vi "ROI group-Remove ROI group.vi"(8 "error in (no error)":errorcluster) -> (0 "error out":errorcluster, 2 "Deleted group setup":T1={"Group number"="", "Group Name"="", "Visibility"=TRUE, "Highlight"=FALSE})   [LabVIEW 2020]
uses:
  Typedefs/Group sel cluster.ctl
  Global variables/gl_Functional Imaging-Global variables.vi
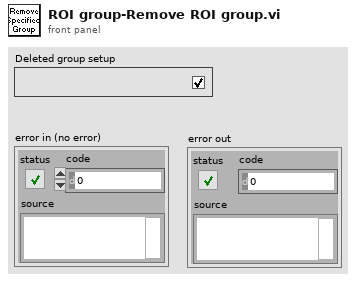
[diagram p1: front panel]
types:
  T1 = typedef "Group sel cluster.ctl" = cluster{"Group number":string, "Group Name":string, "Visibility":bool, "Highlight":bool}
  T2 = typedef "Functional Imging UI Refs.ctl" = cluster{"Menu ref":refnum<k9>, "Image control":refnum<vi>, "VI ref":refnum<vi>, "XGrapher":refnum<vi>, "Smoothing":refnum<vi>, "POI Averaging":refnum<vi>, "Normalize":refnum<vi>, "POI data points in each trial":refnum<vi>, "Channel":refnum<vi>, "Experiment data folder path":refnum<vi>, "[ROI vis]":refnum<vi>, "[Groups] visbl":T3, "Group Name":refnum<vi>, "POI index":refnum<vi>, "Trial No.":refnum<vi>, "Intensity Zoom":refnum<vi>, "Trial Cursor Enabled":refnum<vi>, "Number of Trials (ind 1)":refnum<vi>, "Number of Trials (ind 2)":refnum<vi>, "MiniScans Available":refnum<vi>, "POI Available":refnum<vi>, "Defer graph updates":refnum<vi>, "Waveform selector":refnum<vi>, "#of selected POI":refnum<vi>, "#of selected MiniScans":refnum<vi>, "#of selected groups":refnum<vi>, "Max Z-Projection":refnum<vi>, "Z-Plane Selector":refnum<vi>, "Index of miniscan point to visualise":refnum<vi>, "ROI vis. mode":refnum<vi>, "Total # of points":refnum<vi>, "Index of group clicked on":refnum<vi>, "Pane 1":refnum<vi>, "Pane 2":refnum<vi>, "Pane 3":refnum<vi>, "Pane 4":refnum<vi>, "Pane 5":refnum<vi>, "Pane 6":refnum<vi>, "Deselect all ROI":refnum<vi>, "Deselect all groups":refnum<vi>}
  T3 = typedef "Groups array referecne.ctl" = refnum<vi>
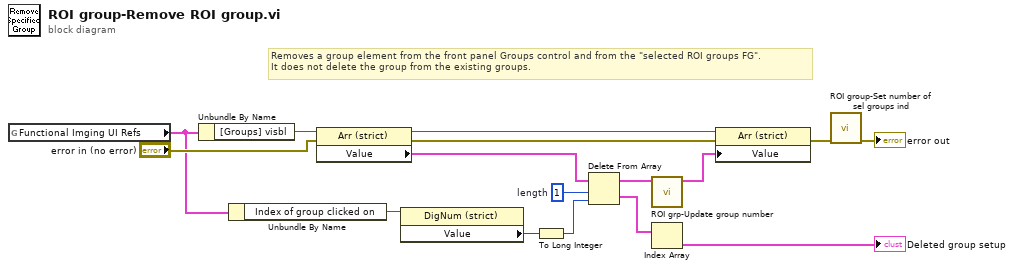
[diagram p0: block diagram]
diagram:
  w11 = 1  # length
  # "Removes a group element from the front panel Groups control and from the \"selected ROI groups FG\".\nIt does not delete the group from the existing groups."
  n1 = global read "gl_Functional Imaging-Global variables.vi" "Functional Imging UI Refs"() -> (w8:T2)
  n2 = Unbundle By Name(w8) -> ("[Groups] visbl"=w15:T3)
  n3 = Unbundle By Name(w8) -> ("Index of group clicked on"=w9:refnum<vi>)
  n4 = property on="Property Node" class="Arr (strict)"(reference=w15, error in="error in (no error)") -> (reference out=w16:T3, error out=w13:errorcluster, "Value"=w12:T1[])
  n5 = property on="Property Node" class="DigNum (strict)"(reference=w9) -> ("Value"=w7:i16)  [unwired: 1 in, 2 out]
  n6 = To Long Integer(number=w7) -> (32bit integer=w10:i32)
  n7 = Delete From Array "Delete From Array"(array=w12, length=w11, index=w10) -> (deleted portion=w2:T1[], array with subset deleted=w4:T1[])
  n8 = call "ROI grp-Update group number.vi"("[Groups]"=w4) -> ("[Groups]"=w3:T1[])  [unwired: 10 in]
  n9 = Index Array(array=w2) -> (element=→"Deleted group setup":T1)  [unwired: 1 in]
  n10 = property on="Property Node" class="Arr (strict)"(reference=w16, error in=w13, "Value"=w3) -> (error out=w6:errorcluster)  [unwired: 1 out]
  n11 = call "ROI group-Set number of sel groups ind.vi"("error in (no error)"=w6) -> ("error out"=→"error out":errorcluster)  [unwired: 10 in]
